vi "Query Signaling RF UL Bandwidth.vi"(8 "error in (no error)":errorcluster, 9 "Cell Name (\"Cell Name\")":string="Cell Name", 11 "VISA resource name":refnum<visa-resource-name>) -> (0 "error out":errorcluster, 2 "UL Bandwidth":i32, 3 "VISA resource name out":refnum<visa-resource-name>)   [LabVIEW 2020, in "Rohde&Schwarz CMWXP NR FR1 Measurement.lvlib"]
doc: "Queries the channel bandwidth for the uplink.\n\nAttribute:\n-\n\nRemote-control command:\n[CONFigure:]SIGNaling:NRADio:CELL:RFSettings:UL:BWIDth?"
uses:
  <instrlib>/Rohde&Schwarz CMWXP NR FR1 Measurement/Rohde&Schwarz CMWXP NR FR1 Measurement.lvlib
  <instrlib>/Rohde&Schwarz CMWXP NR FR1 Measurement/Private/rsidr_core.llb/rsidr_core.lvlib
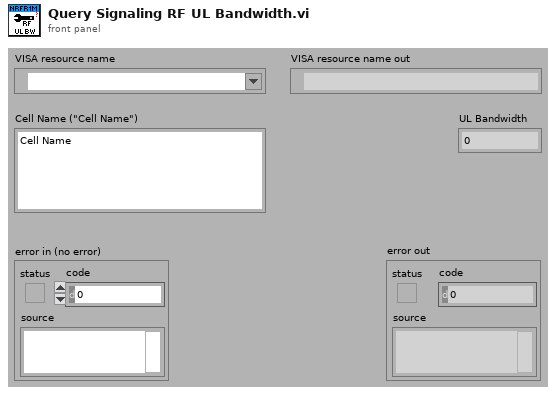
[diagram p1: front panel]
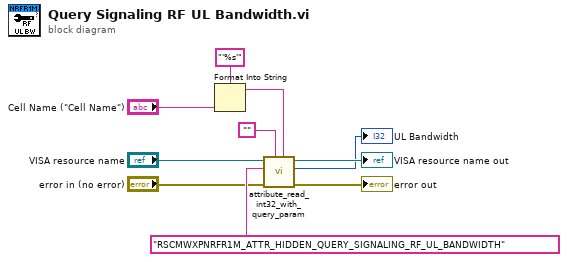
[diagram p0: block diagram]
diagram:
  n1 = Format Into String(format string="'%s'", "Cell Name (\"Cell Name\")") -> (resulting string=w1:string)  [unwired: 2 in, 1 out]
  n2 = call <instrlib>:"attribute_read_int32_with_query_param.vi"("Query Parameter (None)"=w1, "Repeated Capability"="", "error in"="error in (no error)", "Attribute ID"="RSCMWXPNRFR1M_ATTR_HIDDEN_QUERY_SIGNALING_RF_UL_BANDWIDTH", "VISA resource name"="VISA resource name") -> ("error out"=→"error out":errorcluster, "I32 out"=→"UL Bandwidth":i32, "VISA resource name out"=→"VISA resource name out":refnum<visa-resource-name>)  [unwired: 4 in]
